vi "下载HTTP文件.vi"(8 "error in (no error)":errorcluster, 9 "Authentication":cluster{"Username":string, "Password":string}, 11 "Base URL":string) -> (0 "error out":errorcluster, 2 "ok?":bool, 3 "路径":path)   [LabVIEW 2016, in "update.lvlib" / "http client.lvclass"]
uses:
  http client.lvclass
  <vilib>/httpClient/LabVIEWHTTPClient.lvlib
panel:
  out "Content-Length":string
  out "Status Code":u16
  out "HTTP Version":string
  out "Status String":string
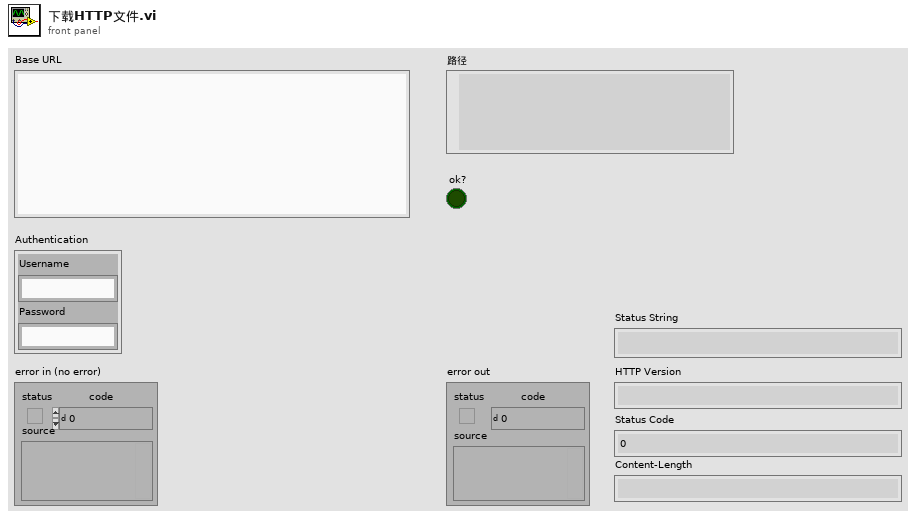
[diagram p1: front panel]
types:
  T1 = typedef "LabVIEWHTTPClient.lvlib/ClientHandle.ctl" = refnum<k1>
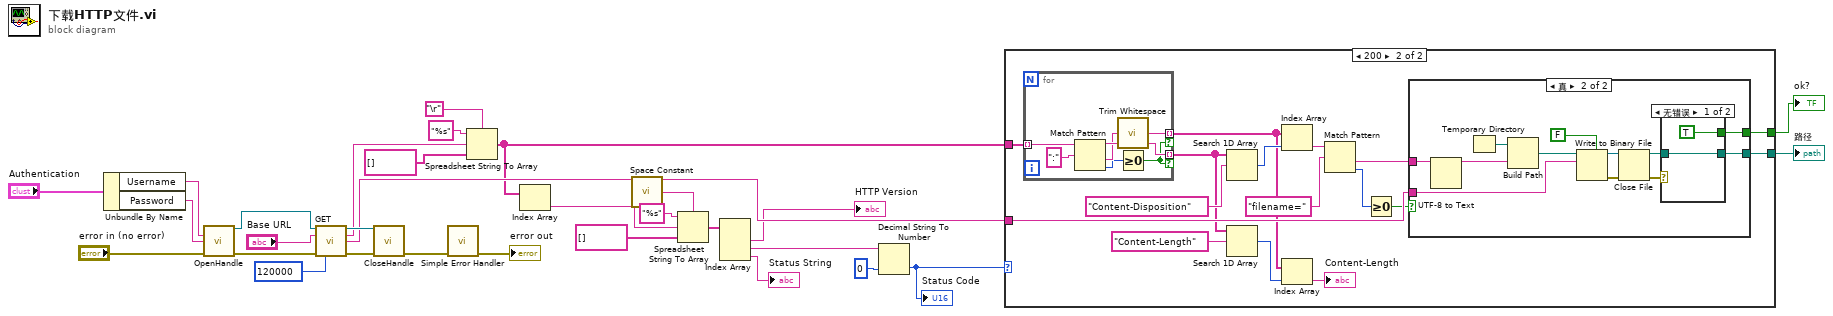
[diagram p0: block diagram]
diagram:
  n1 = Unbundle By Name("Authentication") -> ("Username"=w29:string, "Password"=w28:string)
  n2 = call <vilib>:"OpenHandle.vi"("username"=w29, "password"=w28, "error in (no error)"="error in (no error)") -> ("client handle out"=w27:T1, "error out"=w26:errorcluster)  [unwired: 11 in]
  n3 = call <vilib>:"GET.vi"("client handle"=w27, "url"="Base URL", "error in (no error)"=w26, "timeout (10000)"=120000) -> ("client handle out"=w23:T1, "headers"=w5:string, "body"=w21:string, "error out"=w24:errorcluster)  [unwired: 8 in]
  n4 = call <vilib>:"CloseHandle.vi"("client handle"=w23, "error in (no error)"=w24) -> ("error out"=w3:errorcluster)  [unwired: 13 in]
  n5 = call <vilib>:"Simple Error Handler.vi"("error in (no error)"=w3) -> ("error out"=→"error out":errorcluster)  [unwired: 4 in, 4 out]
  n6 = Spreadsheet String To Array(delimiter (Tab)="\r", format string="%s" ("格式字符串"), spreadsheet string=w5, array type (2D Dbl)=string[] []) -> (array=w4:string[])
  n7 = Index Array(array=w4) -> (element=w17:string)  [unwired: 1 in]
  n8 = call <vilib>:"Space Constant.vi"() -> ("String"=w16:string)
  n9 = Spreadsheet String To Array(delimiter (Tab)=w16, format string="%s" ("格式字符串"), spreadsheet string=w17, array type (2D Dbl)=string[] []) -> (array=w13:string[])
  n10 = Index Array(array=w13) -> (element #1=→"HTTP Version":string, element #2=w11:string, element #3=→"Status String":string)  [unwired: 3 in]
  n11 = Decimal String To Number(string=w11, default (0L)=u16 0 ("默认(0 I32)")) -> (number=w8:u16)  [unwired: 1 in, 1 out]
  "Status Code" <- w8
  n12 = case shown="200" w8 {
    tunnel: w21 -> [_ w44]
    tunnel: w4 -> [_ w43]
    tunnel: [_ w32] -> w2
    tunnel: [_ w31] -> w1
    frame Default {
    }
    frame 200 {
      n13 = for {
        tunnel: w43 -> [w53] mode=indexing
        tunnel: [w51] -> w36 mode=indexing if=w47
        tunnel: [w49] -> w37 mode=indexing if=w47
        n14 = Match Pattern(string=w53, regular expression=":" ("正则表达式")) -> (before substring=w51:string, after substring=w50:string, offset past match=w48:i32)  [unwired: 1 in, 1 out]
        n15 = call <vilib>:"Trim Whitespace.vi"("string"=w50) -> ("trimmed string"=w49:string)  [unwired: 1 in]
        n16 = Greater Or Equal To 0?(x=w48) -> (x >= 0?=w47:bool)
      }
      n17 = Search 1D Array(1D array=w36, element="Content-Disposition" ("Name")) -> (index of element=w41:i32)  [unwired: 1 in]
      n18 = Search 1D Array(1D array=w36, element="Content-Length" ("Name")) -> (index of element=w34:i32)  [unwired: 1 in]
      n19 = Index Array(array=w37, index=w41) -> (element=w40:string)
      n20 = Index Array(array=w37, index=w34) -> (element=→"Content-Length":string)
      n21 = Match Pattern(string=w40, regular expression="filename=" ("正则表达式")) -> (after substring=w46:string, offset past match=w39:i32)  [unwired: 1 in, 2 out]
      n22 = Greater Or Equal To 0?(x=w39) -> (x >= 0?=w38:bool)
      n23 = case shown="真" w38 {
        tunnel: w46 -> [_ w59]
        tunnel: w44 -> [_ w58]
        tunnel: [_ w56] -> w32
        tunnel: [_ w54] -> w31
        frame False {
        }
        frame True {
          n24 = UTF-8 to Text(11:w59) -> (3:w60:string)  [unwired: 2 in, 1 out]
          n25 = Temporary Directory() -> (w63:path)
          n26 = Build Path(base path=w63, name or relative path=w60) -> (appended path=w62:path)
          n27 = Write to Binary File(file (use dialog)=w62, data=w58, 5:FALSE ("预置数组或字符串大小？ (T)")) -> (refnum out=w65:refnum<file>, error out=w64:errorcluster)  [unwired: 3 in, 1 out]
          n28 = Close File(refnum=w65, error in=w64) -> (path=w55:path, error out=w57:errorcluster)
          n29 = case shown="无错误" w57 {
            tunnel: [w67 _] -> w56
            tunnel: w55 -> [w67 _]
            tunnel: [TRUE _] -> w54
            frame No Error {
            }
            frame Error {
            }
          }
        }
      }
    }
  }
  "路径" <- w2
  "ok?" <- w1
